vi "Initialize Controller Class.vi"(0 "Plugin_UI in":refnum<class "Plugin_UI.lvclass">, 11 "error in (no error)":errorcluster) -> (4 "Plugin_UI Out":refnum<class "Plugin_UI.lvclass">, 6 "Plugin_Controller out":refnum<class "Plugin_Controller.lvclass">, 15 "error out":errorcluster)   [LabVIEW 2020, in "Plugin.lvlib" / "Plugin_UI.lvclass"]
doc: "This VI initializes the controller class object with the latest Hardware and Channel information."
uses:
  Plugin_UI.lvclass
  C:/SVN_LabSys/labsys_lvcode/LabSys_SourceCode/builds/Libraries/LabSys Framework.lvlibp/Process/Process/Process.lvclass
  Controller_Class/Plugin_Controller.lvclass
  C:/SVN_LabSys/labsys_lvcode/LabSys_SourceCode/builds/Libraries/LabSys Framework.lvlibp/Configurable Data Node/Configurable Data Node/Configurable Data Node.lvclass
  C:/SVN_LabSys/labsys_lvcode/LabSys_SourceCode/builds/Libraries/LabSys Framework.lvlibp/Data Node/Data Node/Data Node.lvclass
  Plugin_UI.lvclass/Plugin_UI.ctl
  Read Input Channels[].vi
  Read Output Channels[].vi
  Channels/Input Channels/Input Channels.lvclass
  C:/SVN_LabSys/labsys_lvcode/LabSys_SourceCode/Plugin Template/Source/Code/Channels/Plugin_Channels.lvclass
  Channels/Output Channels/Output Channels.lvclass
  builds/Libraries/LabSys Framework.lvlibp/Process/Process/Read Error Manager.vi
  Read Lookup Tables.vi
  Read Scaling Functions.vi
  builds/Libraries/LabSys Framework.lvlibp/Configurable Data Node/Configurable Data Node/Read Module Configuration.vi
  builds/Libraries/LabSys Framework.lvlibp/Data Node/Data Node/Write Module Name.vi
  builds/Libraries/LabSys Framework.lvlibp/Data Node/Data Node/Write Error Manager.vi
  builds/Libraries/LabSys Framework.lvlibp/Configuration Storage/Module Configuration/Set Lookup Tables.vi
  builds/Libraries/LabSys Framework.lvlibp/Configuration Storage/Module Configuration/Set Scaling Functions.vi
  builds/Libraries/LabSys Framework.lvlibp/Configurable Data Node/Configurable Data Node/Write Module Configuration.vi
  builds/Libraries/LabSys Framework.lvlibp/Error Manager/Error Manager/Error Manager.lvclass
  builds/Libraries/LabSys Framework.lvlibp/Configuration Storage/Module Configuration/Module Configuration.lvclass
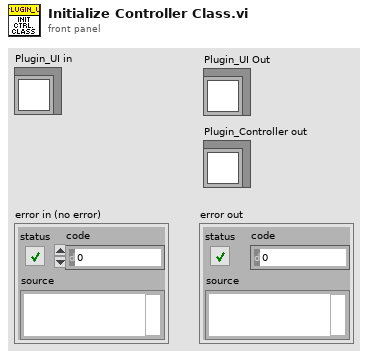
[diagram p1: front panel]
types:
  T1 = typedef "Plugin.lvlib/Plugin_UI.lvclass/UDP Configuration.ctl" = cluster{"Device Port Number":u16, "Device IP":string, "Timeout":i32, "Port Number":u16}
  T2 = typedef "Plugin.lvlib/Plugin_UI.lvclass/Serial Configuration.ctl" = cluster{"VISA":refnum<visa-resource-name>, "Interface Type":T3, "Serial Interface":T4, "Slave Address":u8}
  T3 = typedef "Shared GUI Library.lvlibp/Interface Type.ctl" = u16
  T4 = typedef "Shared GUI Library.lvlibp/Serial Interafce.ctl" = cluster{"Baud Rate":u32, "Data Bits ":u16, "Parity":enum16{"None", "Odd", "Even"}, "Stop Bits":u16}
  T5 = typedef "LabSys Framework.lvlibp/Configuration Storage.lvlib/Test Configuration.lvclass/Table Information.ctl" = cluster{"Name":string, "Lookup Table":dbl[][]}
  T6 = typedef "LabSys Framework.lvlibp/Configuration Storage.lvlib/Test Configuration.lvclass/Function Information.ctl" = cluster{"Name":string, "Expression":string, "Constants":T7[], "Test Data":dbl[][]}
  T7 = typedef "LabSys Framework.lvlibp/Configuration Storage.lvlib/Test Configuration.lvclass/Function Constant Value.ctl" = cluster{"Constant Name":string, "Value":dbl}
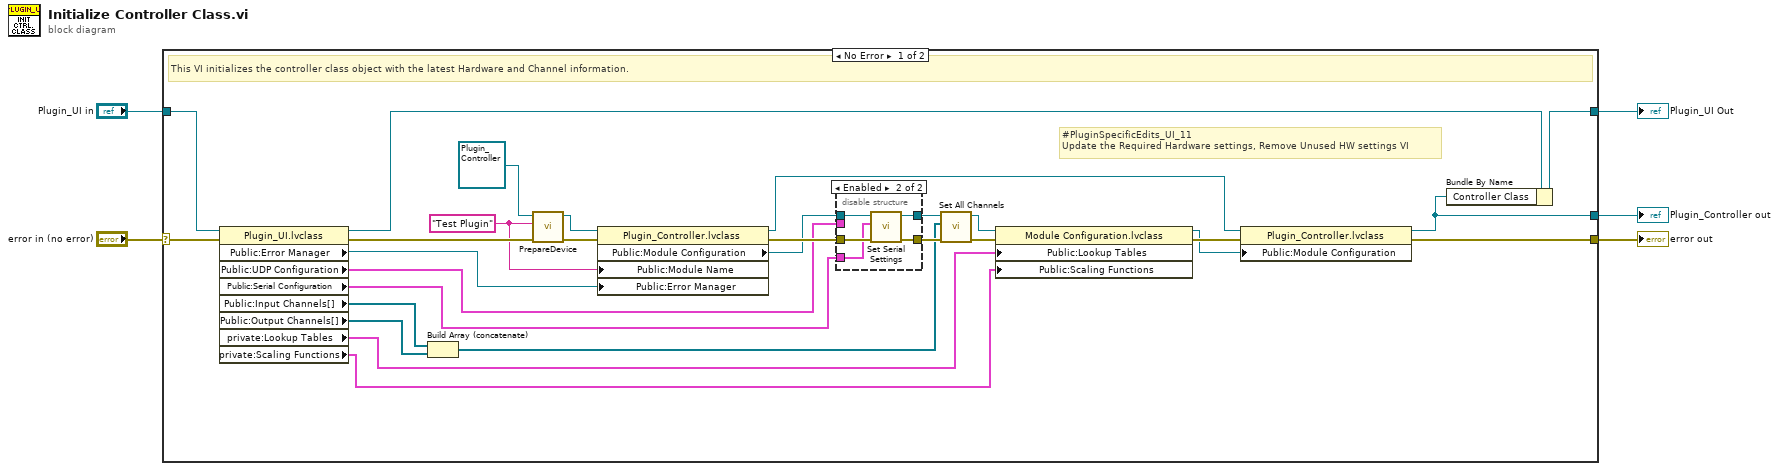
[diagram p0: block diagram]
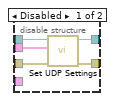
[diagram p2: hidden frame]
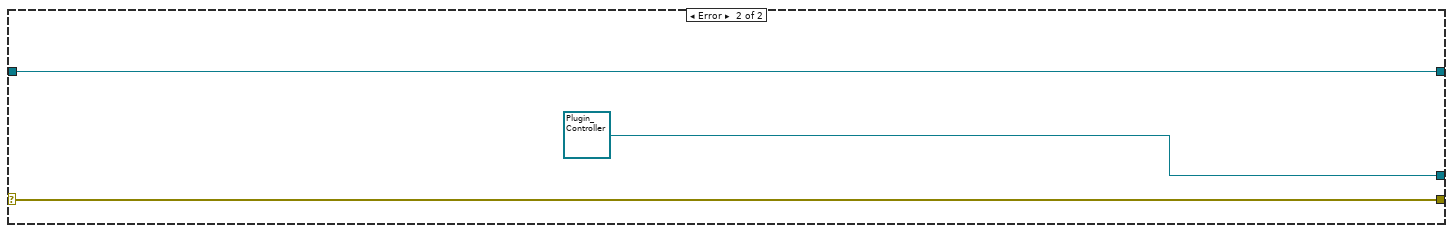
[diagram p3: hidden frame]
diagram:
  n1 = case shown="No Error" "error in (no error)" {
    selector: "error in (no error)" -> [w17 w45]
    tunnel: "Plugin_UI in" -> [w33 w46]
    tunnel: [w15 refnum<class "Plugin_Controller.lvclass"> refnum ("Device Driver out")] -> w4
    tunnel: [w32 w45] -> w3
    tunnel: [w14 w46] -> w2
    frame No Error {
      w13 = "Test Plugin" ("Module Name")
      # "#PluginSpecificEdits_UI_11\nUpdate the Required Hardware settings, Remove Unused HW settings VI"
      # "This VI initializes the controller class object with the latest Hardware and Channel information."
      n2 = property class="Plugin_UI.lvclass"(reference=w33, error in=w17) -> (reference out=w16:refnum<class "Plugin_UI.lvclass">, error out=w24:errorcluster, "Public:Error Manager"=w23:refnum<data-value>, "Public:UDP Configuration"=w22:T1, "Public:Serial Configuration"=w12:T2, "Public:Input Channels[]"=w20:refnum<class "Input Channels.lvclass">[], "Public:Output Channels[]"=w19:refnum<class "Output Channels.lvclass">[], "private:Lookup Tables"=w7:T5[], "private:Scaling Functions"=w6:T6[])
      n3 = Build Array (concatenate)(w20, w19) -> (w18:refnum<class "Plugin_Channels.lvclass">[])
      n4 = call-dynamic "PrepareDevice.vi"("error in"=w24, "Module Name"=w13, "Device Driver in"=refnum<class "Plugin_Controller.lvclass"> refnum ("Plugin.lvlib:Plugin_Controller.lvclass")) -> ("error out"=w25:errorcluster, "Device Driver out"=w21:refnum<class "Plugin_Controller.lvclass">)  [unwired: 7 in]
      n5 = property class="Plugin_Controller.lvclass"(reference=w21, error in=w25, "Public:Module Name"=w13, "Public:Error Manager"=w23) -> (reference out=w28:refnum<class "Plugin_Controller.lvclass">, error out=w30:errorcluster, "Public:Module Configuration"=w26:refnum<class "Module Configuration.lvclass">)
      n6 = disable-structure shown="Enabled" {
        disable-tunnel: w30 -> [w38 w42]
        disable-tunnel: [w37 w43] -> w29
        disable-tunnel: [w36 w40] -> w27
        disable-tunnel: w26 -> [w35 w41]
        disable-tunnel: w22 -> [w34 _]
        disable-tunnel: w12 -> [_ w39]
        frame Disabled {
          n7 = call "Set UDP Settings.vi"("error in (no error)"=w38, "Hardware Configuration"=w34, "Module Configuration"=w35) -> ("error out"=w37:errorcluster, "Module Configuration out"=w36:refnum<class "Module Configuration.lvclass">)  [unwired: 7 in]
        }
        frame Enabled {
          n8 = call "Set Serial Settings.vi"("error IO"=w42, "Serial Configuration"=w39, "Module Configuration"=w41) -> ("error IO out"=w43:errorcluster, "Module Configuration out"=w40:refnum<class "Module Configuration.lvclass">)  [unwired: 7 in]
        }
      }
      n9 = call "Set All Channels.vi"("error in"=w29, "Channels[]"=w18, "Module Configuration in"=w27) -> ("error out"=w10:errorcluster, "Module Configuration out"=w11:refnum<class "Module Configuration.lvclass">)  [unwired: 7 in]
      n10 = property class="Module Configuration.lvclass"(reference=w11, error in=w10, "Public:Lookup Tables"=w7, "Public:Scaling Functions"=w6) -> (reference out=w8:refnum<class "Module Configuration.lvclass">, error out=w9:errorcluster)
      n11 = property class="Plugin_Controller.lvclass"(reference=w28, error in=w9, "Public:Module Configuration"=w8) -> (reference out=w15:refnum<class "Plugin_Controller.lvclass">, error out=w32:errorcluster)
      n12 = Bundle By Name(cluster=w16, "Controller Class"=w15) -> (w14:refnum<class "Plugin_UI.lvclass">)
    }
    frame Error {
    }
  }
  "Plugin_Controller out" <- w4
  "error out" <- w3
  "Plugin_UI Out" <- w2
